vi "Hash Function.vi"(8 "num Buckets":i32, 11 "Constant Name":string) -> (3 "Hash Code":i32)   [LabVIEW 2013]
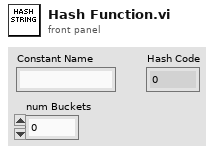
[diagram p1: front panel]
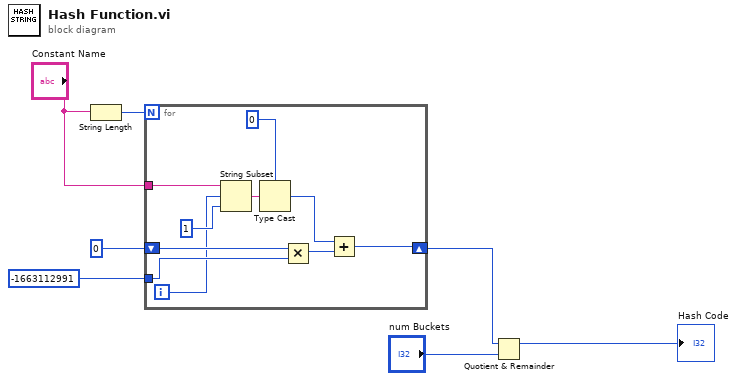
[diagram p0: block diagram]
diagram:
  n1 = String Length(string="Constant Name") -> (length=w4:i32)
  n2 = for {
    N: w4 -> [_]
    tunnel: "Constant Name" -> [w17]
    shift-right: [w9] -> w2
    shift-left: u32 0 ("unsigned 32bit integer") -> [w13]
    tunnel: -1663112991 ("unsigned 32bit integer") -> [w12]
    i -> [w8]
    n3 = String Subset(string=w17, offset (0)=w8, length (rest)=1 ("length (rest)")) -> (substring=w15:string)
    n4 = Type Cast(type=u32 0 ("unsigned 32bit integer"), x=w15) -> (*(type *) &x=w10:u32)
    n5 = Multiply(x=w13, y=w12) -> (x*y=w11:u32)
    n6 = Add(x=w10, y=w11) -> (x+y=w9:u32)
  }
  n7 = Quotient & Remainder(x=w2, y="num Buckets") -> (x-y*floor(x/y)=→"Hash Code":u32)  [unwired: 1 out]
